vi "Init.vi"(5 "PathControl.lvclass":refnum<class "PathControl.lvclass">, 6 "Environmental classes":refnum<class "Instrument.lvclass">[](array[class]), 7 "XML Handler.lvclass":refnum<class "XML Handler.lvclass">, 8 "error in (no error)":errorcluster, 9 "Instruments to Use":T1(array[cluster]), 10 "Device.lvclass":refnum<class "Device.lvclass">, 11 "Switching Times in":refnum<class "Switching Time.lvclass">) -> (0 "error out":errorcluster, 3 "Switching Times out":refnum<class "Switching Time.lvclass">)   [LabVIEW 2020, in "Switching Time.lvclass"]
doc: "Initializes the measurement.\nThis verifies that the instruments are present and adds them into the class data.\nIs also adds the xml handler into the class data."
uses:
  Switching Time.lvclass
  Devices/Device.lvclass
  Instruments/Instrument.lvclass
  XML Handler/XML Handler.lvclass
  Path Control/PathControl.lvclass
  Controls/Init States.ctl
  Instruments/Oscilloscope/Oscilloscope.lvclass
  Instruments/Spectrum Analyzer/Spectrum Analyzer.lvclass
  Instruments/Signal Generator/Signal Generator.lvclass
  C:/Sandbox/RF Bench/Source Code/WiSpry Test Framework/Instruments/Instrument.lvclass
  Measurement.lvclass
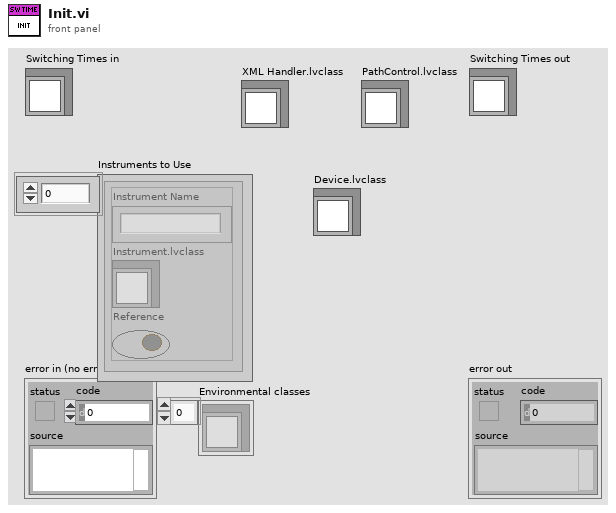
[diagram p1: front panel]
types:
  T1 = cluster{"Instrument Name":string, "Instrument.lvclass":refnum<class "Instrument.lvclass">, "Reference":bool}[]
  T2 = typedef "Measurement.lvclass/Init States.ctl" = enum16{"Verify instruments", "Init Parameters", "Init Instruments", "Add Device", "Init Device", "Create test in XML", "Set path", "Done"}
  T3 = typedef "Switching Time.lvclass/Method.ctl" = enum16{"Oscilloscope", "Spectrum Analyzer"}
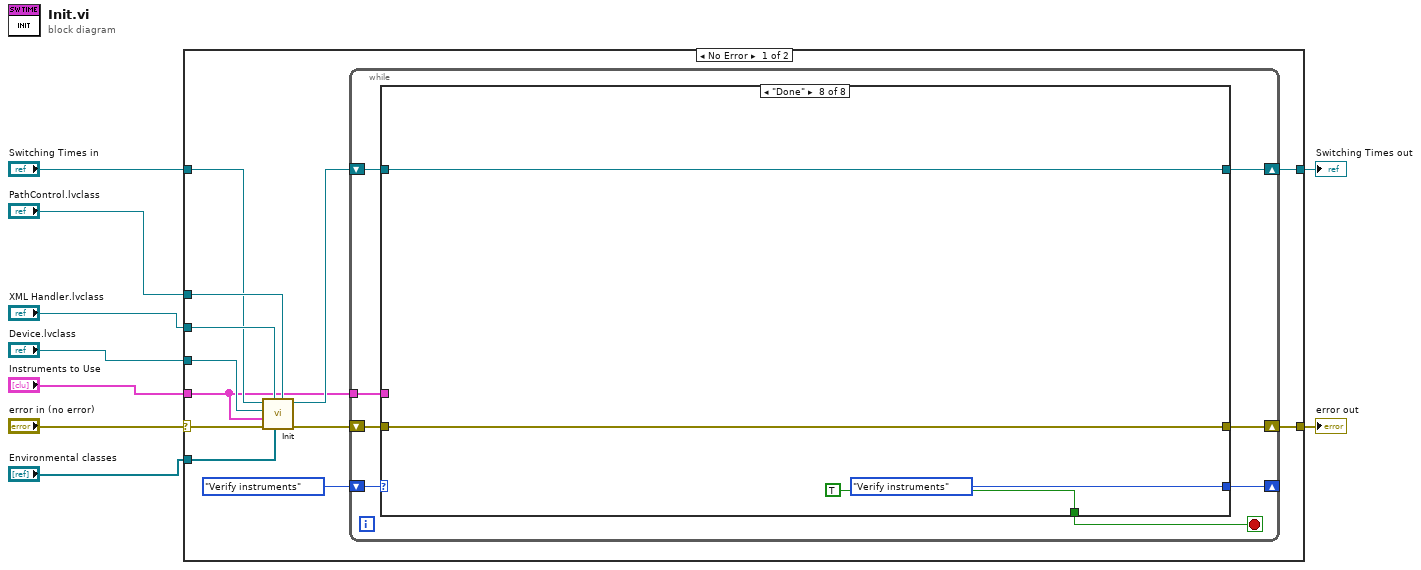
[diagram p0: block diagram]
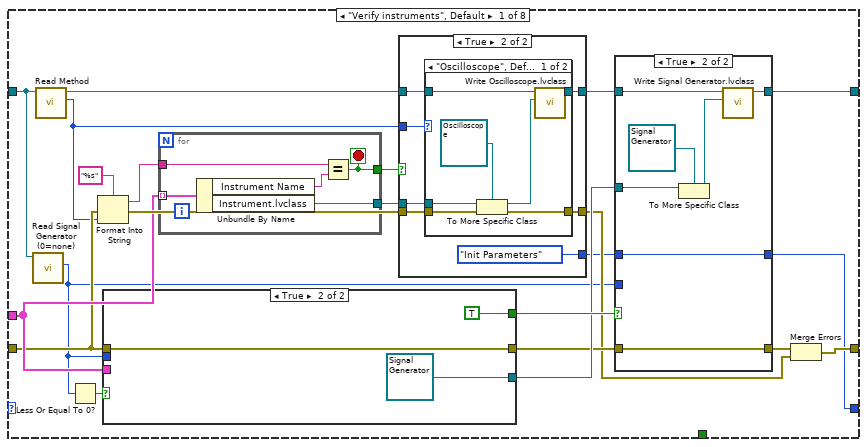
[diagram p2: hidden frame]
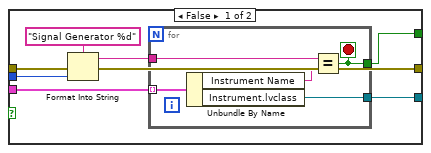
[diagram p3: hidden frame]
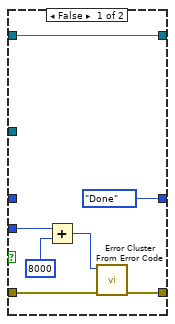
[diagram p4: hidden frame]
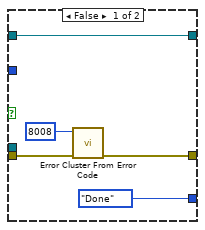
[diagram p5: hidden frame]
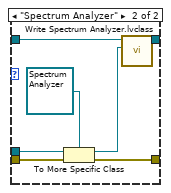
[diagram p6: hidden frame]
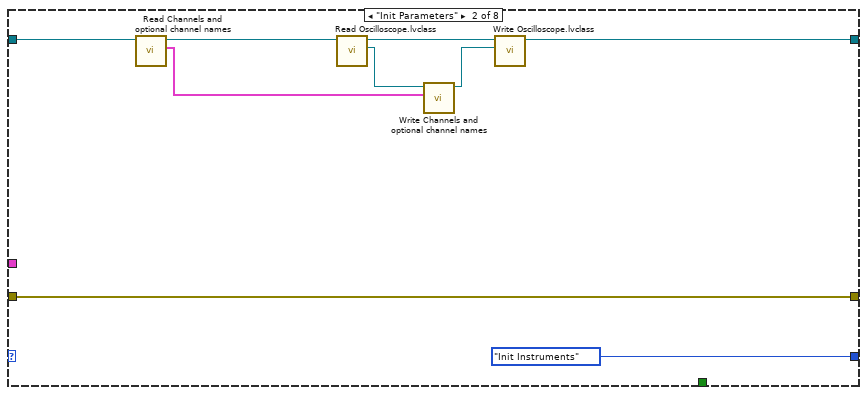
[diagram p7: hidden frame]
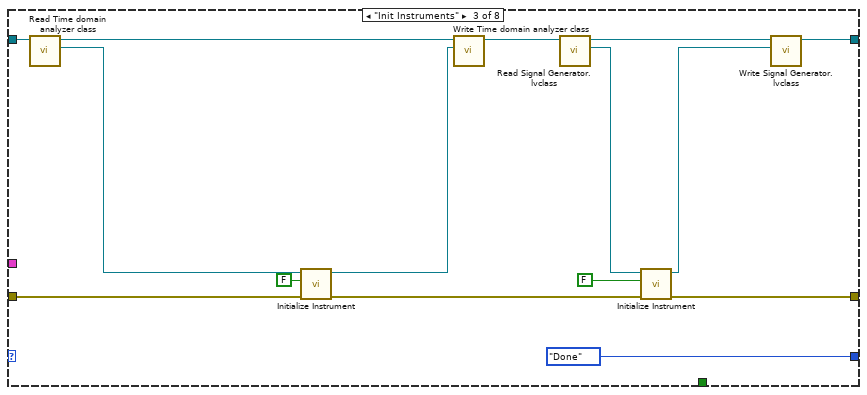
[diagram p8: hidden frame]
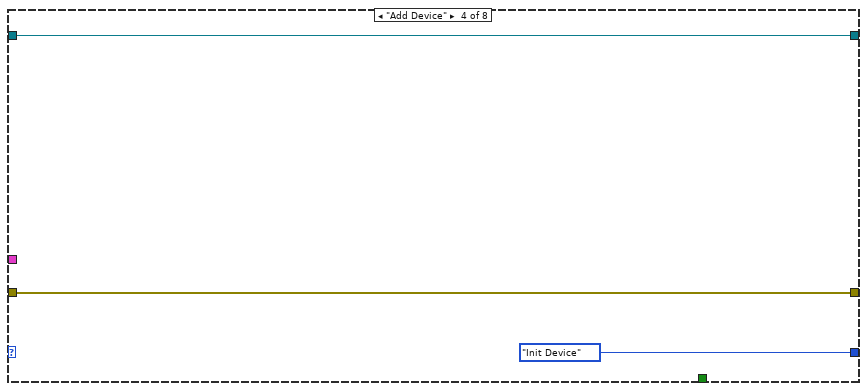
[diagram p9: hidden frame]
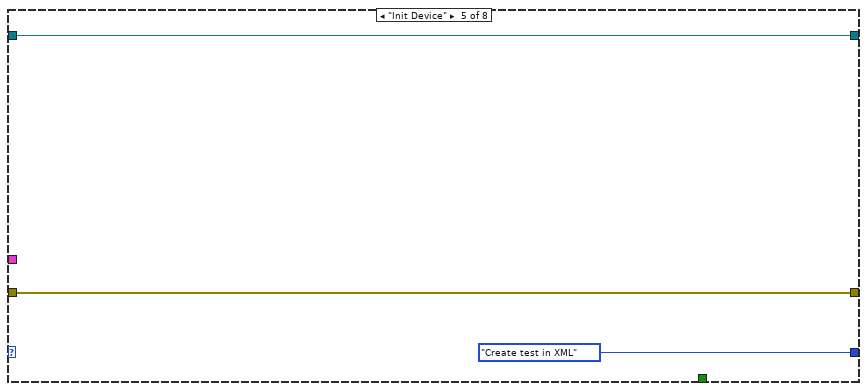
[diagram p10: hidden frame]
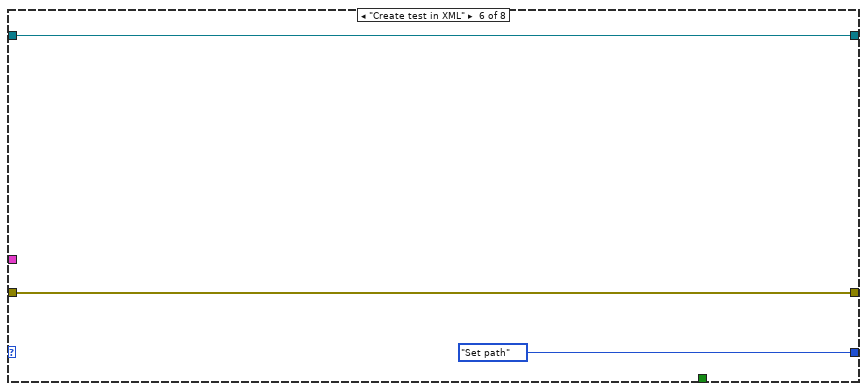
[diagram p11: hidden frame]
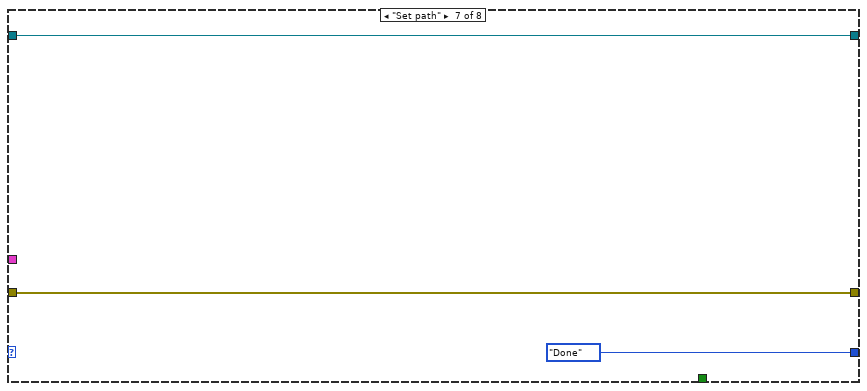
[diagram p12: hidden frame]
diagram:
  n1 = case shown="No Error" "error in (no error)" {
    selector: "error in (no error)" -> [w18 w153]
    tunnel: "PathControl.lvclass" -> [w21 _]
    tunnel: "Environmental classes" -> [w20 _]
    tunnel: "XML Handler.lvclass" -> [w19 _]
    tunnel: "Instruments to Use" -> [w10 _]
    tunnel: "Device.lvclass" -> [w17 _]
    tunnel: "Switching Times in" -> [w16 w154]
    tunnel: [w13 w153] -> w9
    tunnel: [w12 w154] -> w8
    frame No Error {
      n2 = call-parent "Init.vi"("PathControl.lvclass"=w21, "Environmental classes"=w20, "XML Handler.lvclass"=w19, "error in (no error)"=w18, "Instruments to Use"=w10, "Device.lvclass"=w17, "Measurements in"=w16) -> ("error out"=w14:errorcluster, "Measurements out"=w11:refnum<class "Switching Time.lvclass">)  [unwired: 3 in]
      n3 = while {
        shift-right: [w27] -> w13
        shift-left: w14 -> [w28]
        shift-right: [w26] -> w12
        shift-left: w11 -> [w25]
        shift-right: [w23] -> _
        shift-left: Init_States."Verify instruments" ("Init States") -> [w29]
        tunnel: w10 -> [w22]
        stop <- w24 stop-if-true
        n4 = case shown="\"Done\"" w29 {
          tunnel: w28 -> [w44 w121 w127 w139 w142 w145 w148 w152]
          tunnel: [w34 w121 w125 w139 w142 w145 w148 w152] -> w27
          tunnel: [w38 w114 w122 w138 w141 w144 w147 w151] -> w26
          tunnel: w25 -> [w45 w115 w135 w138 w141 w144 w147 w151]
          tunnel: [_ _ _ _ _ _ _ TRUE] -> w24
          tunnel: [w31 Init_States."Init Instruments" ("Init States") Init_States."Done" ("Init States") Init_States."Init Device" ("Init States") Init_States."Create test in XML" ("Init States") Init_States."Set path" ("Init States") Init_States."Done" ("Init States") Init_States."Verify instruments" ("Init States")] -> w23
          tunnel: w22 -> [w46 _ _ _ _ _ _ _]
          frame "Verify instruments", Default {
            n5 = call-dynamic "Read Signal Generator (0=none).vi"("Switching Time in"=w45) -> ("Signal Generator (0=none)"=w30:i32)  [unwired: 9 in, 1 out]
            n6 = call-dynamic "Read Method.vi"("Switching Time in"=w45) -> ("Method"=w42:T3, "Switching Time out"=w50:refnum<class "Switching Time.lvclass">)  [unwired: 9 in]
            n7 = Less Or Equal To 0?(x=w30) -> (x <= 0?=w33:bool)
            n8 = Format Into String(format string="%s", error in=w44, w42) -> (resulting string=w48:string, error out=w47:errorcluster)  [unwired: 1 in]
            n9 = case shown="True" w33 {
              tunnel: w46 -> [w59 _]
              tunnel: w30 -> [w57 _]
              tunnel: w44 -> [w56 w65]
              tunnel: [w54 TRUE] -> w43
              tunnel: [w53 refnum<class "Signal Generator.lvclass"> refnum ("Signal Generator.lvclass")] -> w40
              tunnel: [w52 w65] -> w37
              frame False {
                n10 = Format Into String(format string="Signal Generator %d", error in=w56, w57) -> (resulting string=w55:string, error out=w52:errorcluster)  [unwired: 1 in]
                n11 = for {
                  tunnel: w59 -> [w64] mode=indexing
                  tunnel: w55 -> [w62]
                  tunnel: [w61] -> w54
                  tunnel: [w60] -> w53
                  stop <- w61 stop-if-true
                  n12 = Unbundle By Name(w64) -> ("Instrument Name"=w63:string, "Instrument.lvclass"=w60:refnum<class "Instrument.lvclass">)
                  n13 = Equal?(x=w62, y=w63) -> (x = y?=w61:bool)
                }
              }
              frame True {
              }
            }
            n14 = for {
              tunnel: w46 -> [w112] mode=indexing
              tunnel: w48 -> [w110]
              tunnel: [w109] -> w41
              tunnel: [w108] -> w51
              stop <- w109 stop-if-true
              n15 = Unbundle By Name(w112) -> ("Instrument Name"=w111:string, "Instrument.lvclass"=w108:refnum<class "Instrument.lvclass">)
              n16 = Equal?(x=w110, y=w111) -> (x = y?=w109:bool)
            }
            n17 = case shown="True" w41 {
              tunnel: w50 -> [w86 w92]
              tunnel: w51 -> [_ w93]
              tunnel: [w86 w90] -> w39
              tunnel: w47 -> [w85 w89]
              tunnel: [w83 w88] -> w35
              tunnel: [Init_States."Done" ("Init States") Init_States."Init Parameters" ("Init States")] -> w32
              tunnel: w42 -> [_ w87]
              frame False {
                n18 = call <vilib>:"Error Cluster From Error Code.vi"("error in (no error)"=w85, "error code (0)"=8008) -> ("error out"=w83:errorcluster)  [unwired: 7 in]
              }
              frame True {
                n19 = case shown="\"Oscilloscope\", Default" w87 {
                  tunnel: w93 -> [w100 w107]
                  tunnel: w92 -> [w99 w106]
                  tunnel: [w98 w105] -> w90
                  tunnel: w89 -> [w95 w103]
                  tunnel: [w94 w102] -> w88
                  frame "Oscilloscope", Default {
                    n20 = To More Specific Class(target class=refnum<class "Oscilloscope.lvclass"> refnum ("Oscilloscope.lvclass"), reference=w100, error in=w95) -> (specific class reference=w96:refnum<class "Oscilloscope.lvclass">, error out=w94:errorcluster)
                    n21 = call-dynamic "Write Oscilloscope.lvclass.vi"("Oscilloscope.lvclass"=w96, "Switching Time in"=w99) -> ("Switching Time out"=w98:refnum<class "Switching Time.lvclass">)  [unwired: 9 in]
                  }
                  frame "Spectrum Analyzer" {
                    n22 = To More Specific Class(target class=refnum<class "Spectrum Analyzer.lvclass"> refnum ("Spectrum Analyzer.lvclass"), reference=w107, error in=w103) -> (specific class reference=w104:refnum<class "Spectrum Analyzer.lvclass">, error out=w102:errorcluster)
                    n23 = call-dynamic "Write Spectrum Analyzer.lvclass.vi"("Spectrum Analyzer.lvclass"=w104, "Switching Time in"=w106) -> ("Switching Time out"=w105:refnum<class "Switching Time.lvclass">)  [unwired: 9 in]
                  }
                }
              }
            }
            n24 = case shown="True" w43 {
              tunnel: w39 -> [w74 w78]
              tunnel: w40 -> [_ w81]
              tunnel: [w74 w77] -> w38
              tunnel: w37 -> [w73 w80]
              tunnel: [w72 w80] -> w36
              tunnel: w32 -> [_ w75]
              tunnel: [Init_States."Done" ("Init States") w75] -> w31
              tunnel: w30 -> [w70 _]
              frame False {
                n25 = Add(x=w70, y=8000 ("error code (0)")) -> (x+y=w68:i32)
                n26 = call <vilib>:"Error Cluster From Error Code.vi"("error in (no error)"=w73, "error code (0)"=w68) -> ("error out"=w72:errorcluster)  [unwired: 7 in]
              }
              frame True {
                n27 = To More Specific Class(target class=refnum<class "Signal Generator.lvclass"> refnum ("Signal Generator.lvclass"), reference=w81) -> (specific class reference=w76:refnum<class "Signal Generator.lvclass">)  [unwired: 1 in, 1 out]
                n28 = call-dynamic "Write Signal Generator.lvclass.vi"("Signal Generator.lvclass"=w76, "Switching Time in"=w78) -> ("Switching Time out"=w77:refnum<class "Switching Time.lvclass">)  [unwired: 9 in]
              }
            }
            n29 = Merge Errors(w36, w35) -> (w34:errorcluster)
          }
          frame "Init Parameters" {
            n30 = call-dynamic "Read Channels and optional channel names.vi"("Switching Time in"=w115) -> ("Channels and optional channel names"=w113:cluster{"Enabled":bool, "Channel name":string}[], "Switching Time out"=w116:refnum<class "Switching Time.lvclass">)  [unwired: 9 in]
            n31 = call-dynamic "Read Oscilloscope.lvclass.vi"("Switching Time in"=w116) -> ("Oscilloscope.lvclass"=w119:refnum<class "Oscilloscope.lvclass">, "Switching Time out"=w117:refnum<class "Switching Time.lvclass">)  [unwired: 9 in]
            n32 = call-dynamic "Write Channels and optional channel names.vi"("Channels and optional channel names"=w113, "Oscilloscope in"=w119) -> ("Oscilloscope out"=w118:refnum<class "Oscilloscope.lvclass">)  [unwired: 9 in]
            n33 = call-dynamic "Write Oscilloscope.lvclass.vi"("Oscilloscope.lvclass"=w118, "Switching Time in"=w117) -> ("Switching Time out"=w114:refnum<class "Switching Time.lvclass">)  [unwired: 9 in]
          }
          frame "Init Instruments" {
            n34 = call-dynamic "Read Time domain analyzer class.vi"("Switching Time in"=w135) -> ("Instrument.lvclass"=w134:refnum<class "Instrument.lvclass">, "Switching Time out"=w130:refnum<class "Switching Time.lvclass">)  [unwired: 9 in]
            n35 = call-dynamic "Initialize Instrument.vi"("error in (no error)"=w127, "Reset"=FALSE, "Instrument in"=w134) -> ("error out"=w126:errorcluster, "Instrument out"=w128:refnum<class "Instrument.lvclass">)  [unwired: 7 in]
            n36 = call-dynamic "Write Time domain analyzer class.vi"("Instrument.lvclass"=w128, "Switching Time in"=w130) -> ("Switching Time out"=w129:refnum<class "Switching Time.lvclass">)  [unwired: 9 in]
            n37 = call-dynamic "Read Signal Generator.lvclass.vi"("Switching Time in"=w129) -> ("Signal Generator.lvclass"=w131:refnum<class "Signal Generator.lvclass">, "Switching Time out"=w123:refnum<class "Switching Time.lvclass">)  [unwired: 9 in]
            n38 = call-dynamic "Initialize Instrument.vi"("error in (no error)"=w126, "Reset"=FALSE, "Instrument in"=w131) -> ("error out"=w125:errorcluster, "Instrument out"=w124:refnum<class "Signal Generator.lvclass">)  [unwired: 7 in]
            n39 = call-dynamic "Write Signal Generator.lvclass.vi"("Signal Generator.lvclass"=w124, "Switching Time in"=w123) -> ("Switching Time out"=w122:refnum<class "Switching Time.lvclass">)  [unwired: 9 in]
          }
          frame "Add Device" {
          }
          frame "Init Device" {
          }
          frame "Create test in XML" {
          }
          frame "Set path" {
          }
          frame "Done" {
          }
        }
      }
    }
    frame Error {
    }
  }
  "error out" <- w9
  "Switching Times out" <- w8
